vi "2013_02_18 Pre-Clinical Main.vi"() -> ()   [LabVIEW 2013]
uses:
  Pre-Clinical Type Def.ctl
  <vilib>/DAQmx/write.llb/DAQmx Write (Analog 1D DBL NChan 1Samp).vi
  <vilib>/DAQmx/write.llb/DAQmx Write (Counter Time 1Chan 1Samp).vi
  <vilib>/DAQmx/read.llb/DAQmx Read (Analog 1D Wfm NChan NSamp).vi
  <vilib>/DAQmx/miscellaneous.llb/DAQmx Fill In Error Info.vi
  <resource>/objmgr/daqmx.rc
  <vilib>/measure/NI_MABase.lvlib
panel:
  in  "PWM %":dbl(slide)=100.0 min=0.0 max=100.0 step=5.0 scale=0.0..100.0 scale format="%#.2g"
  in  "Off (s)":u32
  in  "On (s)":u32=60
  in  "PWM On":bool
  in  "Comments":string
  in  "Test ID and Serial #":string="default"
  in  "Motor":T1(ring)
  in  "Clear":bool
  in  "Record":bool=TRUE
  out "Error":bool
  out "XY Graph 3":cluster{"Array":dbl[], "Array":dbl[]}[](graph)
  in  "X axis":u16(ring)=5 items=["Elapsed Time (s)"=0, "Source Current (A)"=10, "Supply (V)"=4, "Supply Power (W)"=11, "RMS Current (A) 1"=1, "RMS Voltage (V) 1"=2, "Electrical Power (W)"=6, "ESC Efficiency (%)"=12, "Torque (mNm)"=5, "RPM"=3, "Mechanical Power(W)"=7, "Motor Efficiency (%)"=8]
  in  "Y axis":u16(ring)=3 items=["Elapsed Time (s)"=0, "Source Current (A)"=10, "Supply (V)"=4, "Supply Power (W)"=11, "RMS Current (A) 1"=1, "RMS Voltage (V) 1"=2, "Electrical Power (W)"=6, "ESC Efficiency (%)"=12, "Torque (mNm)"=5, "RPM"=3, "Mechanical Power(W)"=7, "Motor Efficiency (%)"=8]
  out "TotalSampPerChanAcquired":dbl
  out "AvailSampPerChan":u32
  out "XY Graph 2":cluster{"Array":dbl[], "Array":dbl[]}[](graph)
  out "Single Motor 2":waveform(dbl)[](graph)
  in  "Waveform":bool
  out "XY Graph":cluster{"Array":dbl[], "Array":dbl[]}(graph)
  out "error out":errorcluster
  in  "File Path":path=path "C:/Users/Bullpen/Dropbox/Procyrion/Quality System/Hardware/Motors/Quality Results/.lvm"
  in  "Motor 1":T2 {"ESC Eff" format="%#_3g%%"; "Supply (W)" format="%.3f"; "Mechanical (W)" format="%.3f"; "Motor Eff" format="%#_3g%%"; "Electrical (W)" format="%.3f"; "Torque (mNm)" format="%.3f"; "Time" format="%<%H:%M:%S>t"; "Supply (V)" format="%.2f"}
  out "loop time (ms)":u32
  in  "stop":bool
  # "Stopped"
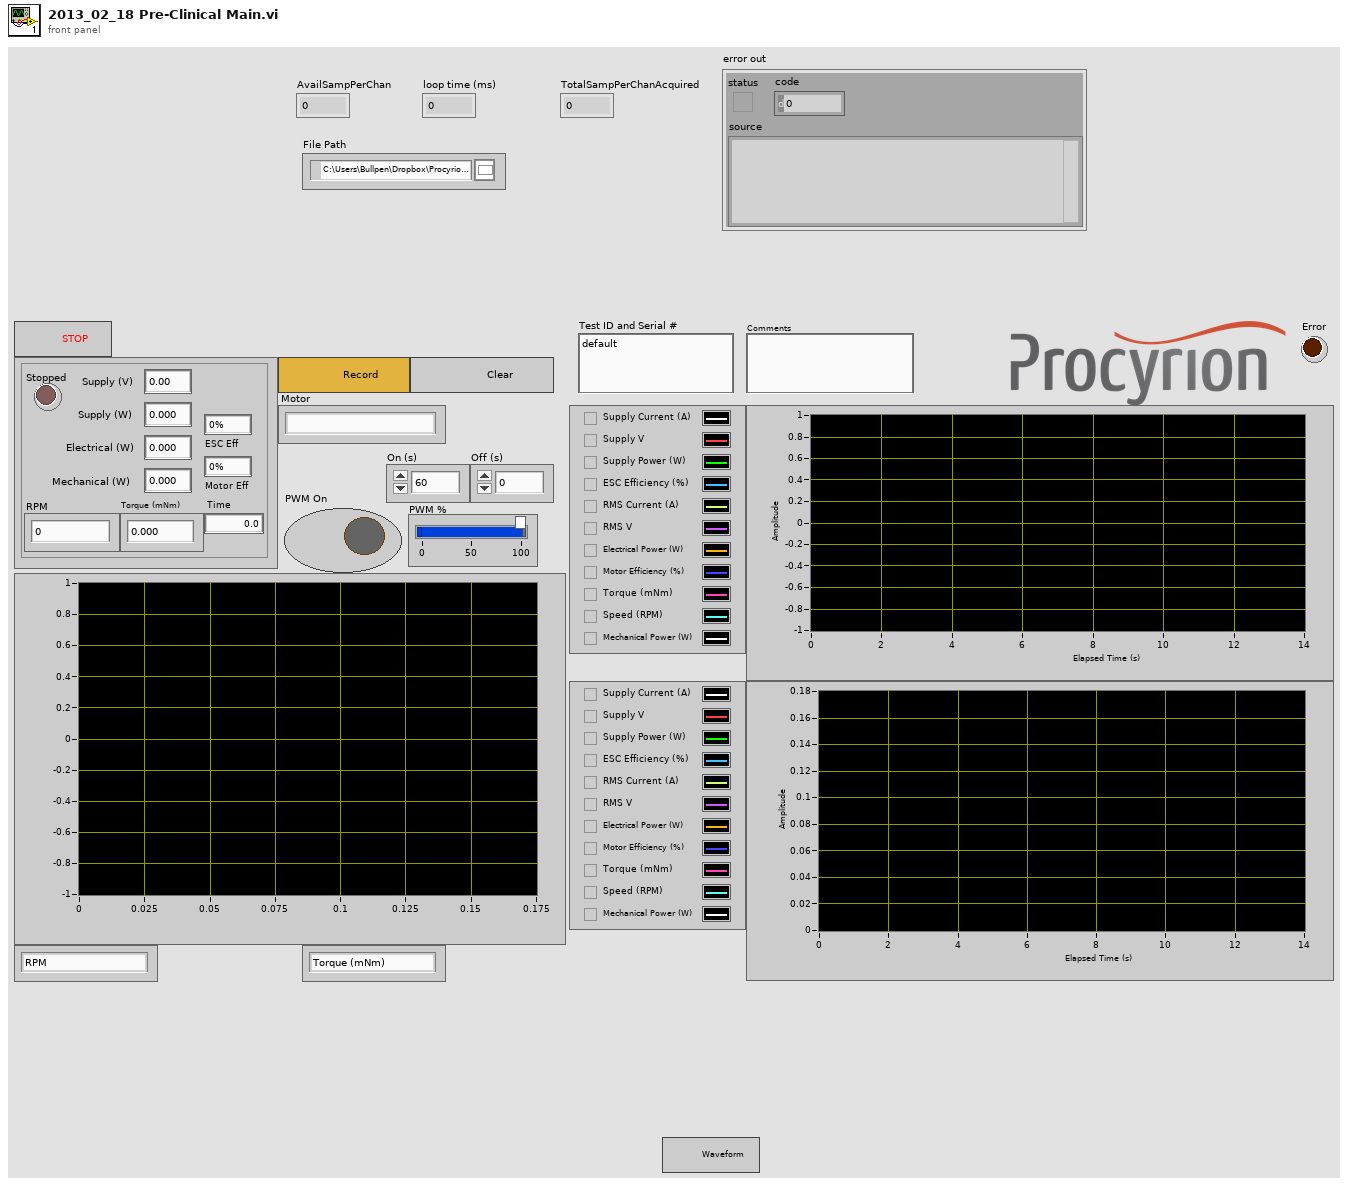
[diagram p1: front panel]
types:
  T1 = enum16{"", "Maxon EC6 6V", "Maxon EC4 6V", "FH 0620 6V", "FH 0620 12V", "FH 0427 6V K2540"}
  T2 = typedef "Pre-Clinical Type Def.ctl" = cluster{"Fail":bool, "RPM":u64, "Supply (V)":dbl, "Time":dbl, "Counter":dbl, "Torque (mNm)":dbl, "Electrical (W)":dbl, "Motor Eff":dbl, "Mechanical (W)":dbl, "Supply (W)":dbl, "ESC Eff":dbl}
  T3 = cluster{"Test ID and Serial #":string, "Comments":string, "Motor":enum16{"", "Maxon EC6 6V", "Maxon EC4 6V", "FH 0620 6V", "FH 0620 12V", "FH 0427 6V K2540"}, "Record":bool, "Clear":bool}
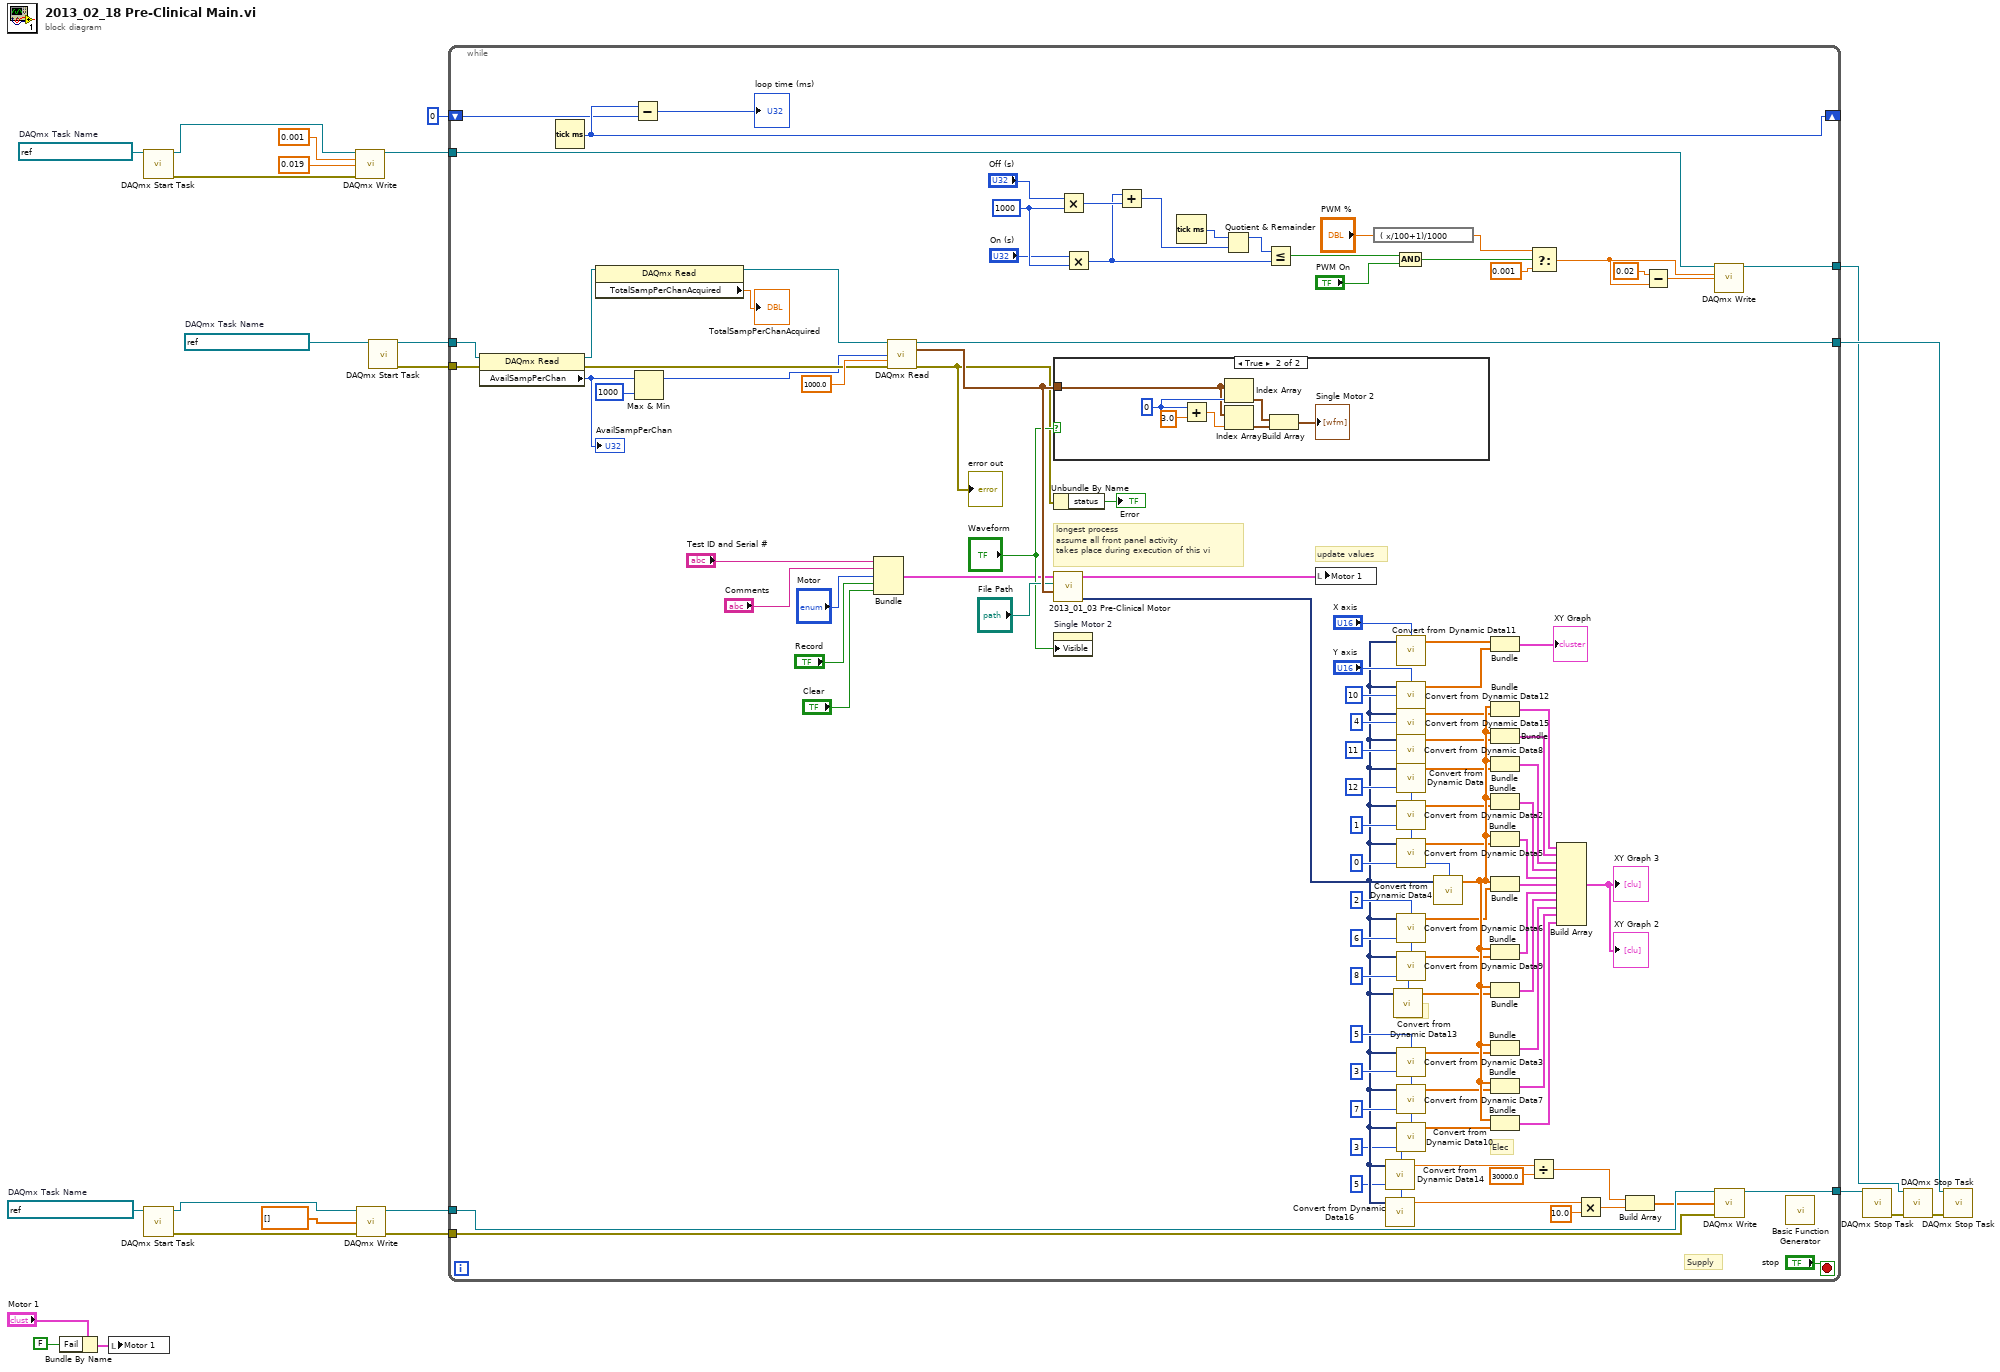
[diagram p0: block diagram]
diagram:
  w8 = refnum<k21> "Pre-Clinical ADI Out"  # DAQmx Task Name
  w22 = refnum<k21> "Pre-Clinical PWM"  # DAQmx Task Name
  w9 = refnum<k21> "Pre-Clinical Acquire"  # DAQmx Task Name
  n1 = Bundle By Name(cluster="Motor 1", "Fail"=FALSE) -> (w10:T2)
  n2 = local write "Motor 1"(w10) -> ()
  n3 = call <vilib>:"DAQmx Start Task.vi"("task/channels in"=w22) -> ("task out"=w20:refnum<k21>, "error out"=w19:errorcluster)  [unwired: 13 in]
  n4 = call <vilib>:"DAQmx Start Task.vi"("task/channels in"=w8) -> ("task out"=w7:refnum<k21>, "error out"=w6:errorcluster)  [unwired: 13 in]
  n5 = call-poly <vilib>:"DAQmx Write.vi"("task/channels in"=w20, "high time"=0.001 ("data"), "low time"=0.019 ("data"), "error in"=w19) -> ("task out"=w21:refnum<k21>)  [unwired: 9 in, 2 out]
  n6 = call-poly <vilib>:"DAQmx Write.vi"("task/channels in"=w7, "data"=dbl[] [], "error in"=w6) -> ("task out"=w5:refnum<k21>, "error out"=w3:errorcluster)  [unwired: 10 in, 1 out]
  n7 = call <vilib>:"DAQmx Start Task.vi"("task/channels in"=w9) -> ("task out"=w24:refnum<k21>, "error out"=w13:errorcluster)  [unwired: 13 in]
  n8 = while {
    tunnel: w24 -> [w102]
    tunnel: [w118] -> w23
    tunnel: w13 -> [w100]
    shift-right: [w123] -> _
    shift-left: u32 0 ("millisecond timer value") -> [w122]
    tunnel: w21 -> [w120]
    tunnel: [w119] -> w18
    tunnel: w5 -> [w65]
    tunnel: w3 -> [w58]
    tunnel: [w57] -> w2
    stop <- "stop" stop-if-true
    w33 = u32 1000 ("y")
    # "Mech"
    # "Elec"
    # "Supply"
    # "update values"
    # "longest process\nassume all front panel activity\ntakes place during execution of this vi"
    n9 = property class="DAQmx Read"(reference=w102, error in=w100) -> (reference out=w98:refnum<k21>, error out=w99:errorcluster, "AvailSampPerChan"=w94:u32)
    "AvailSampPerChan" <- w94
    n10 = Tick Count (ms)() -> (millisecond timer value=w123:u32)
    n11 = property class="DAQmx Read"(reference=w98) -> (reference out=w97:refnum<k21>, "TotalSampPerChanAcquired"=→"TotalSampPerChanAcquired":dbl)  [unwired: 1 in, 1 out]
    n12 = Subtract(x=w123, y=w122) -> (x-y=→"loop time (ms)":u32)
    n13 = Max & Min(x=w94, y=1000 ("number of samples per channel")) -> (max(x,y)=w93:u32)  [unwired: 1 out]
    n14 = Bundle("Test ID and Serial #"="Test ID and Serial #", "Comments"="Comments", "Motor"="Motor", "Record"="Record", "Clear"="Clear") -> (w26:T3)  [unwired: 1 in]
    n15 = call-poly <vilib>:"DAQmx Read.vi"("task/channels in"=w97, "number of samples per channel"=w93, "timeout"=1000.0, "error in"=w99) -> ("task out"=w118:refnum<k21>, "data"=w117:waveform(dbl)[], "error out"=w66:errorcluster)  [unwired: 9 in]
    "error out" <- w66
    n16 = case shown="True" "Waveform" {
      tunnel: w117 -> [_ w129]
      frame False {
      }
      frame True {
        w130 = 0 ("index")
        n17 = Add(x=w130, y=3.0) -> (x+y=w128:dbl)
        n18 = Index Array(array=w129, index=w130) -> (element=w127:waveform(dbl))
        n19 = Index Array(array=w129, index=w128) -> (element=w126:waveform(dbl))
        n20 = Build Array(w127, w126) -> (→"Single Motor 2":waveform(dbl)[])
      }
    }
    n21 = Unbundle By Name(w66) -> ("status"=→"Error":bool)
    n22 = call "2013_01_03 Pre-Clinical Motor.vi"("data"=w117, "File Path"="File Path", "cluster"=w26) -> ("Final Out"=w61:dynamicdata, "Motor Typedef Out"=w49:T2)  [unwired: 7 in]
    n23 = property on="Single Motor 2" class="WFGraph (strict)"("Visible"="Waveform") -> ()  [unwired: 2 in, 2 out]
    n24 = Multiply(x="Off (s)", y=w33) -> (x*y=w35:u32)
    n25 = Multiply(x="On (s)", y=w33) -> (x*y=w30:u32)
    n26 = Add(x=w30, y=w35) -> (x+y=w34:u32)
    n27 = Tick Count (ms)() -> (millisecond timer value=w37:u32)
    n28 = Quotient & Remainder(x=w37, y=w34) -> (x-y*floor(x/y)=w36:u32)  [unwired: 1 out]
    n29 = Less Or Equal?(x=w36, y=w30) -> (x <= y?=w29:bool)
    n30 = local write "Motor 1"(w49) -> ()
    n31 = expression code="( x/100+1)/1000"("PWM %") -> (w38:dbl)
    n32 = call "Convert from Dynamic Data14"("Dynamic Data Type"=w61, "Channel"=3) -> ("Scalar"=w55:dbl)  [unwired: 2 in]
    n33 = call "Convert from Dynamic Data16"("Dynamic Data Type"=w61, "Channel"=5) -> ("Scalar"=w50:dbl)  [unwired: 2 in]
    n34 = call "Convert from Dynamic Data13"("Dynamic Data Type"=w61, "Channel"=8) -> ("Array"=w68:dbl[])  [unwired: 2 in]
    n35 = And(x=w29, y="PWM On") -> (x .and. y?=w27:bool)
    n36 = call "Convert from Dynamic Data11"("Dynamic Data Type"=w61, "Channel"="X axis") -> ("Array"=w90:dbl[])  [unwired: 2 in]
    n37 = call "Convert from Dynamic Data12"("Dynamic Data Type"=w61, "Channel"="Y axis") -> ("Array"=w91:dbl[])  [unwired: 2 in]
    n38 = call "Convert from Dynamic Data15"("Dynamic Data Type"=w61, "Channel"=10) -> ("Array"=w88:dbl[])  [unwired: 2 in]
    n39 = call "Convert from Dynamic Data8"("Dynamic Data Type"=w61, "Channel"=4) -> ("Array"=w74:dbl[])  [unwired: 2 in]
    n40 = call "Convert from Dynamic Data"("Dynamic Data Type"=w61, "Channel"=11) -> ("Array"=w73:dbl[])  [unwired: 2 in]
    n41 = call "Convert from Dynamic Data2"("Dynamic Data Type"=w61, "Channel"=12) -> ("Array"=w72:dbl[])  [unwired: 2 in]
    n42 = call "Convert from Dynamic Data5"("Dynamic Data Type"=w61, "Channel"=1) -> ("Array"=w71:dbl[])  [unwired: 2 in]
    n43 = call "Convert from Dynamic Data6"("Dynamic Data Type"=w61, "Channel"=2) -> ("Array"=w70:dbl[])  [unwired: 2 in]
    n44 = call "Convert from Dynamic Data9"("Dynamic Data Type"=w61, "Channel"=6) -> ("Array"=w87:dbl[])  [unwired: 2 in]
    n45 = call "Convert from Dynamic Data3"("Dynamic Data Type"=w61, "Channel"=5) -> ("Array"=w63:dbl[])  [unwired: 2 in]
    n46 = call "Convert from Dynamic Data7"("Dynamic Data Type"=w61, "Channel"=3) -> ("Array"=w62:dbl[])  [unwired: 2 in]
    n47 = call "Convert from Dynamic Data10"("Dynamic Data Type"=w61, "Channel"=7) -> ("Array"=w69:dbl[])  [unwired: 2 in]
    n48 = call "Convert from Dynamic Data4"("Dynamic Data Type"=w61, "Channel"=0) -> ("Array"=w89:dbl[])  [unwired: 2 in]
    n49 = Bundle("Array"=w90, "Array"=w91) -> (→"XY Graph":cluster{"Array":dbl[], "Array":dbl[]})  [unwired: 1 in]
    n50 = Bundle("Array"=w89, "Array"=w88) -> (w106:cluster{"Array":dbl[], "Array":dbl[]})  [unwired: 1 in]
    n51 = Bundle("Array"=w89, "Array"=w74) -> (w107:cluster{"Array":dbl[], "Array":dbl[]})  [unwired: 1 in]
    n52 = Bundle("Array"=w89, "Array"=w73) -> (w108:cluster{"Array":dbl[], "Array":dbl[]})  [unwired: 1 in]
    n53 = Bundle("Array"=w89, "Array"=w72) -> (w109:cluster{"Array":dbl[], "Array":dbl[]})  [unwired: 1 in]
    n54 = Bundle("Array"=w89, "Array"=w71) -> (w110:cluster{"Array":dbl[], "Array":dbl[]})  [unwired: 1 in]
    n55 = Bundle("Array"=w89, "Array"=w70) -> (w111:cluster{"Array":dbl[], "Array":dbl[]})  [unwired: 1 in]
    n56 = Bundle("Array"=w89, "Array"=w87) -> (w112:cluster{"Array":dbl[], "Array":dbl[]})  [unwired: 1 in]
    n57 = Bundle("Array"=w89, "Array"=w68) -> (w113:cluster{"Array":dbl[], "Array":dbl[]})  [unwired: 1 in]
    n58 = Bundle("Array"=w89, "Array"=w63) -> (w115:cluster{"Array":dbl[], "Array":dbl[]})  [unwired: 1 in]
    n59 = Bundle("Array"=w89, "Array"=w62) -> (w114:cluster{"Array":dbl[], "Array":dbl[]})  [unwired: 1 in]
    n60 = Bundle("Array"=w89, "Array"=w69) -> (w104:cluster{"Array":dbl[], "Array":dbl[]})  [unwired: 1 in]
    n61 = Divide(x=w55, y=30000.0) -> (x/y=w54:dbl)
    n62 = Select(t=w38, s=w27, f=0.001) -> (s? t:f=w40:dbl)
    n63 = Build Array(w106, w107, w108, w109, w110, w111, w112, w113, w115, w114, w104) -> (→"XY Graph 2" →"XY Graph 3":cluster{"Array":dbl[], "Array":dbl[]}[])
    n64 = Multiply(x=w50, y=10.0) -> (x*y=w51:dbl)
    n65 = Build Array(w54, w51) -> (w53:dbl[])
    n66 = Subtract(x=0.02 ("y"), y=w40) -> (x-y=w41:dbl)
    n67 = call-poly <vilib>:"DAQmx Write.vi"("task/channels in"=w120, "high time"=w40, "low time"=w41) -> ("task out"=w119:refnum<k21>)  [unwired: 10 in, 2 out]
    n68 = call-poly <vilib>:"DAQmx Write.vi"("task/channels in"=w65, "data"=w53, "error in"=w58) -> ("task out"=w57:refnum<k21>)  [unwired: 10 in, 2 out]
    n69 = call <vilib>:"Basic Function Generator.vi"() -> ()  [unwired: 9 in, 3 out]
  }
  n70 = call <vilib>:"DAQmx Stop Task.vi"("task/channels in"=w2) -> ("error out"=w1:errorcluster)  [unwired: 13 in, 1 out]
  n71 = call <vilib>:"DAQmx Stop Task.vi"("task/channels in"=w18, "error in"=w1) -> ("error out"=w17:errorcluster)  [unwired: 12 in, 1 out]
  n72 = call <vilib>:"DAQmx Stop Task.vi"("task/channels in"=w23, "error in"=w17) -> ()  [unwired: 12 in, 2 out]
